vi "CONDOM.vi"() -> ()   [LabVIEW 2018]
panel:
  out "Tank":dbl(slide) scale=0.0..10.0
  in  "Voltage":dbl(knob) scale=0.0..2000.0
  out "Voltage":dbl
  out "Level Lubricante":dbl(slide) scale=0.0..100.0
  in  "Level Lubricante":dbl(knob) scale=0.0..100.0
  out "Lubricante":bool
  in  "Lubricante":bool
  out "MaxLub":bool
  out "MinLub":bool
  out "Lubricante":dbl(slide) scale=0.0..10.0
  out "Voltaje":bool
  in  "Voltaje":bool
  out "LSecado":bool
  in  "Secado":bool
  out "MaxTal":bool
  out "MinTal":bool
  out "LLavado":bool
  in  "Lavado":bool
  out "LTalco":bool
  in  "Talco":bool
  out "Tanque de Talco":dbl(slide) scale=0.0..10.0
  out "MinC":bool
  out "MaxC":bool
  out "Tanque de Condones":dbl(slide) scale=0.0..10.0
  out "L Quitar":bool
  in  "Quitar":bool
  out "T Vulcanus":dbl(slide) scale=0.0..100.0
  in  "T Vulcanus":dbl(knob) scale=0.0..100.0
  out "L Vulcano":bool
  in  "Vulcanizacion":bool
  out "L Bordes":bool
  in  "Bordes":bool
  out "L F2":bool
  in  "Fase2":bool
  out "L F1":bool
  in  "Fase1":bool
  out "LClean":bool
  in  "Clean":bool
  in  "Secadora por Calor":bool
  out "L Seco":bool
  out "T Sec":dbl(slide) scale=0.0..100.0
  in  "T Sec":dbl(knob) scale=0.0..100.0
  out "L Lab":bool
  in  "Lavado":bool
  out "min Lab":bool
  out "Max Lab":bool
  out "Min Bat":bool
  out "Max Bat":bool
  out "min Mad":bool
  out "Max Mad":bool
  out "min4":bool
  out "Max4":bool
  out "min3":bool
  out "Max3":bool
  out "min Cal":bool
  out "Max Cal":bool
  out "min Mez":bool
  out "Max Mez":bool
  out "min2":bool
  out "Max2":bool
  out "min1":bool
  out "Max1":bool
  in  "stop":bool
  out "L Cal":bool
  in  "Calentador":bool
  out "CAL":dbl(slide) scale=0.0..150.0
  in  "CAL":dbl(knob) scale=0.0..150.0
  out "Valvula Calentador":bool
  out "Lavado":dbl(slide) scale=0.0..10.0
  out "Calentador":dbl(slide) scale=0.0..10.0
  out "Valvula HOT":bool
  out "Valvula Madu":bool
  out "Valvula Mix":bool
  out "Valvula Agua":bool
  out "Valvula Quimicos":bool
  out "Valvula Jabon":bool
  out "Valvula Latex Normal":bool
  out "Valvula Latex Sensitive":bool
  out "TEMP":dbl(slide) scale=0.0..200.0
  in  "TEMP":dbl(knob) scale=0.0..200.0
  out "L Batea":bool
  out "L Madu":bool
  out "L Mix":bool
  in  "Batea":bool
  in  "Maduracion":bool
  in  "Mezcladora":bool
  out "L Latex S":bool
  out "L Latex N":bool
  out "L AguaQJ":bool
  in  "Latex Sensitive":bool
  in  "Latex Normal":bool
  in  "accion":bool
  out "Maduracion":dbl(slide) scale=0.0..50.0
  out "Max":bool
  out "min":bool
  out "Latex Sensitive":dbl(slide) scale=0.0..10.0
  out "Batea":dbl(slide) scale=0.0..50.0
  out "Mezcladora":dbl(slide) scale=0.0..50.0
  out "Agua":dbl(slide) scale=0.0..20.0
  out "Latex Normal":dbl(slide) scale=0.0..10.0
  out "Jabon":dbl(slide) scale=0.0..10.0
  out "Quimicos":dbl(slide) scale=0.0..10.0
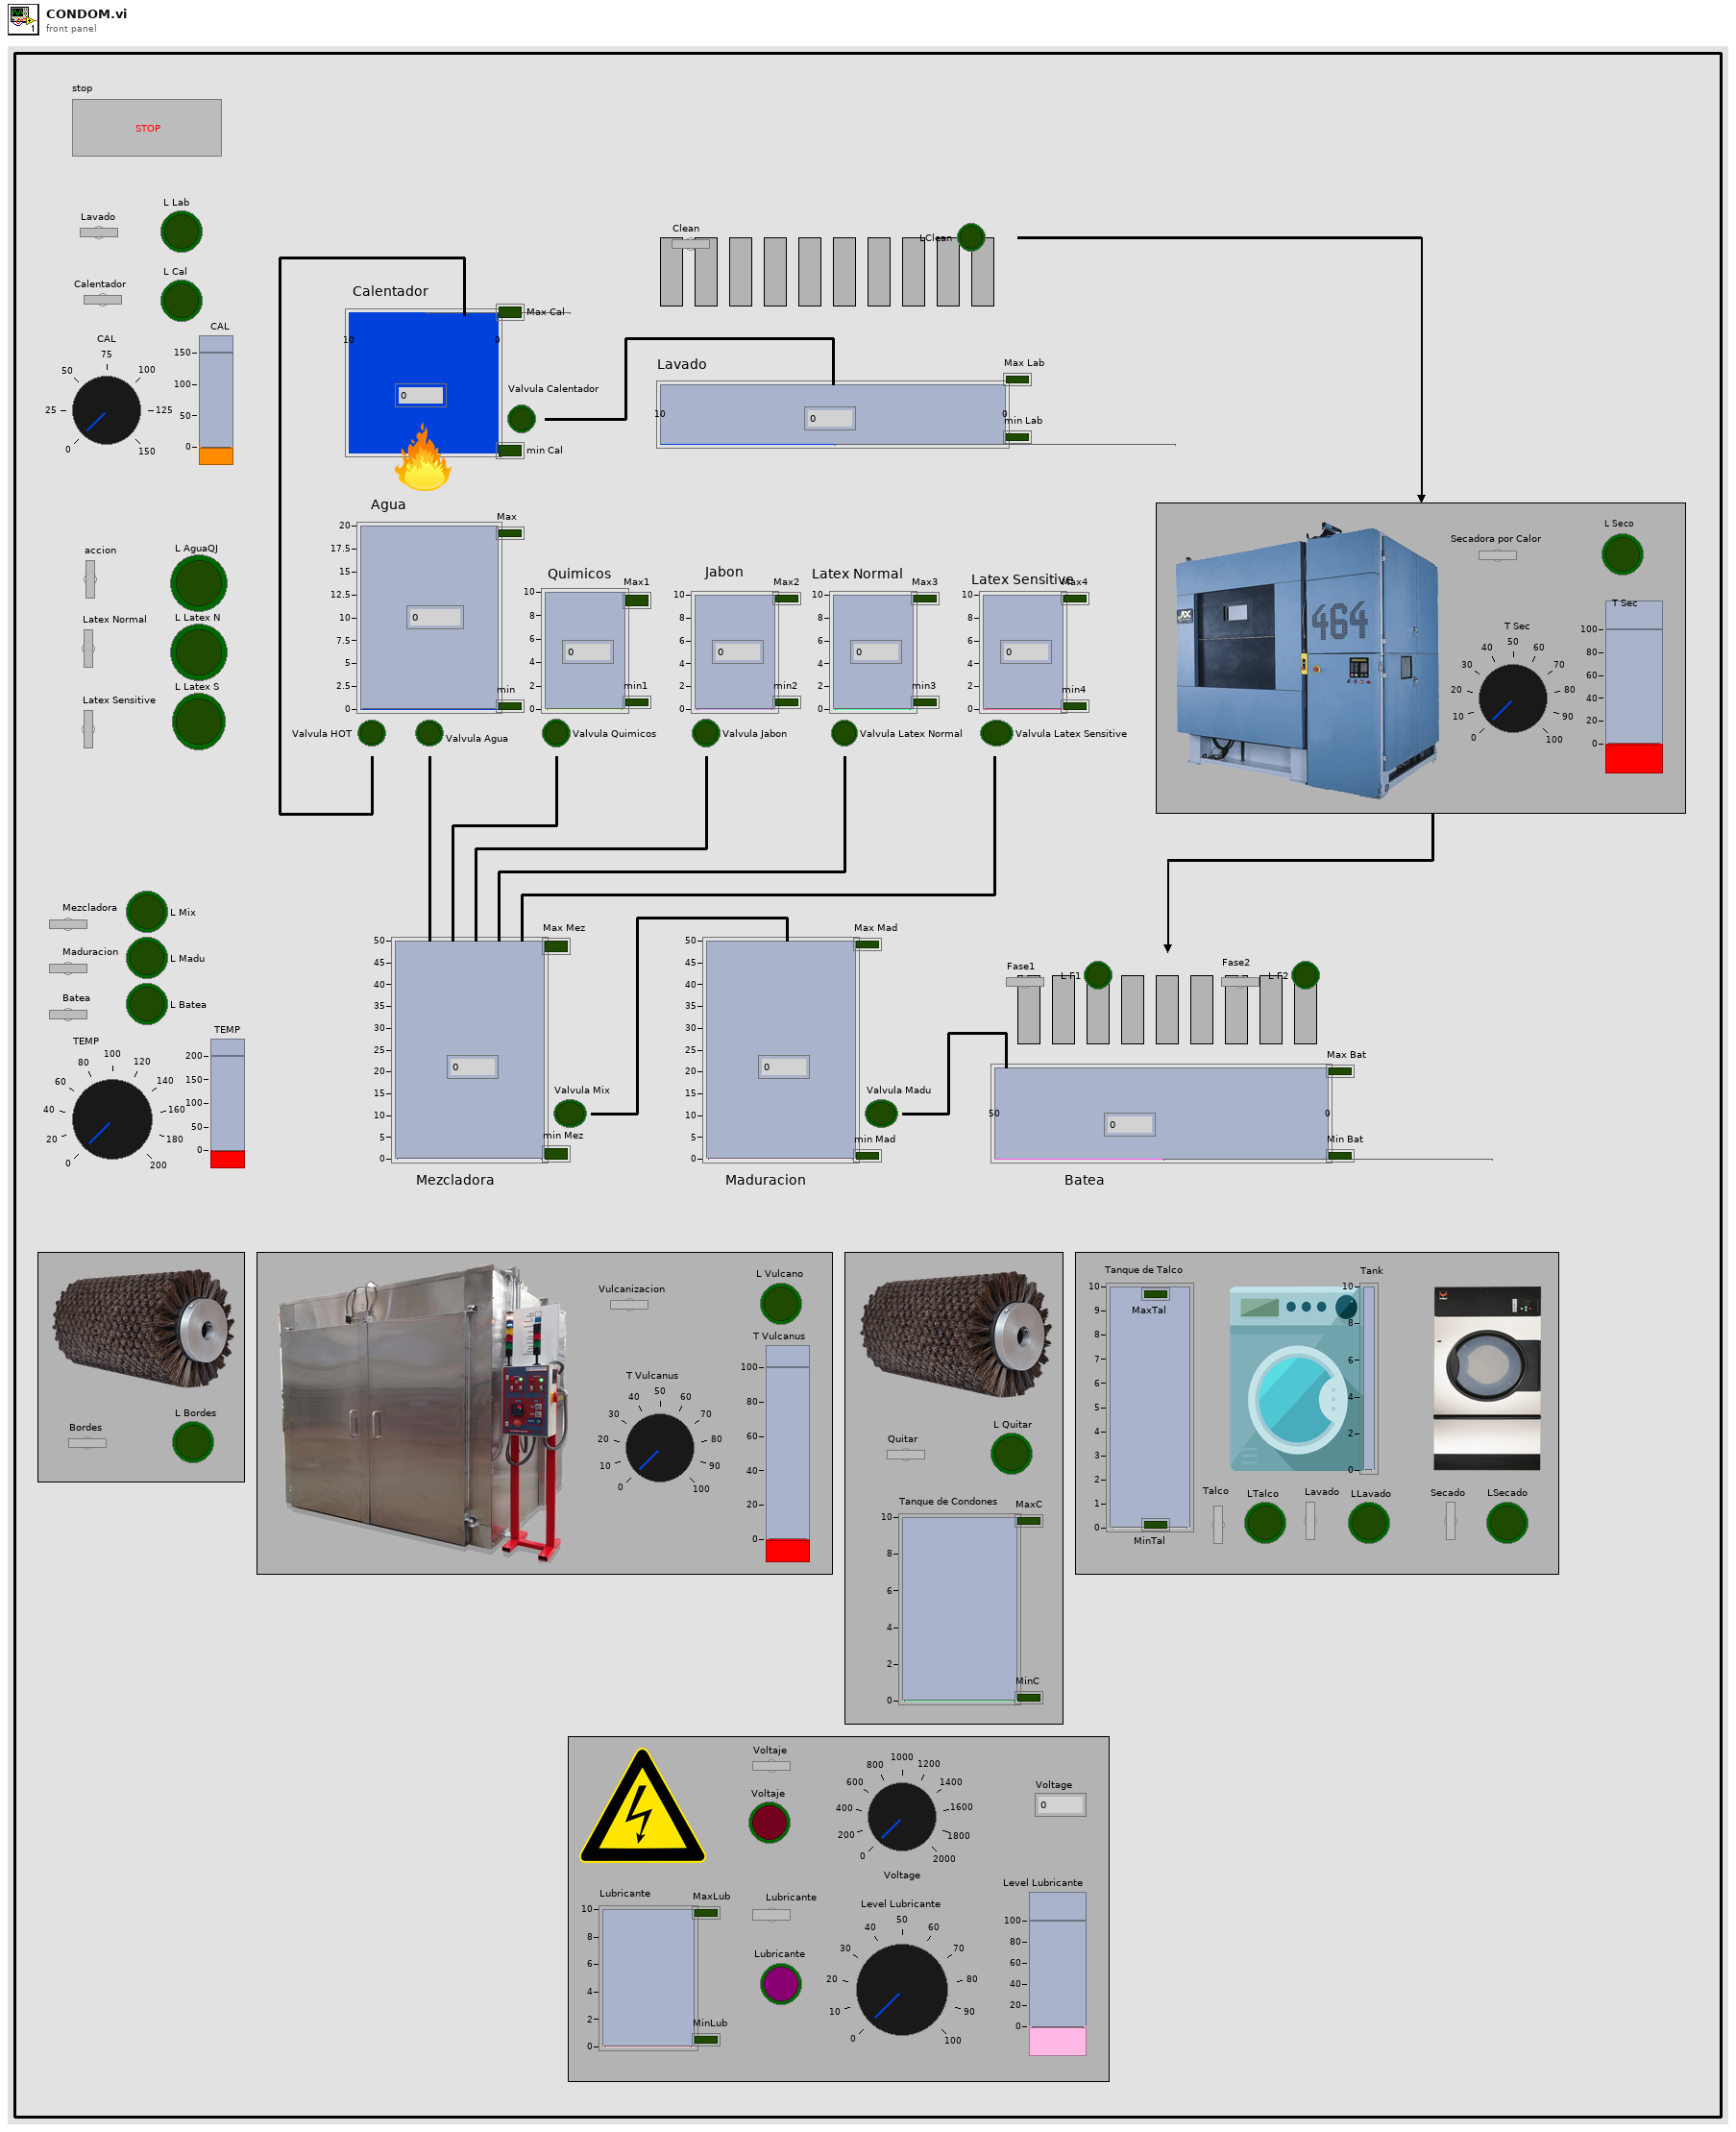
[diagram p1: front panel]
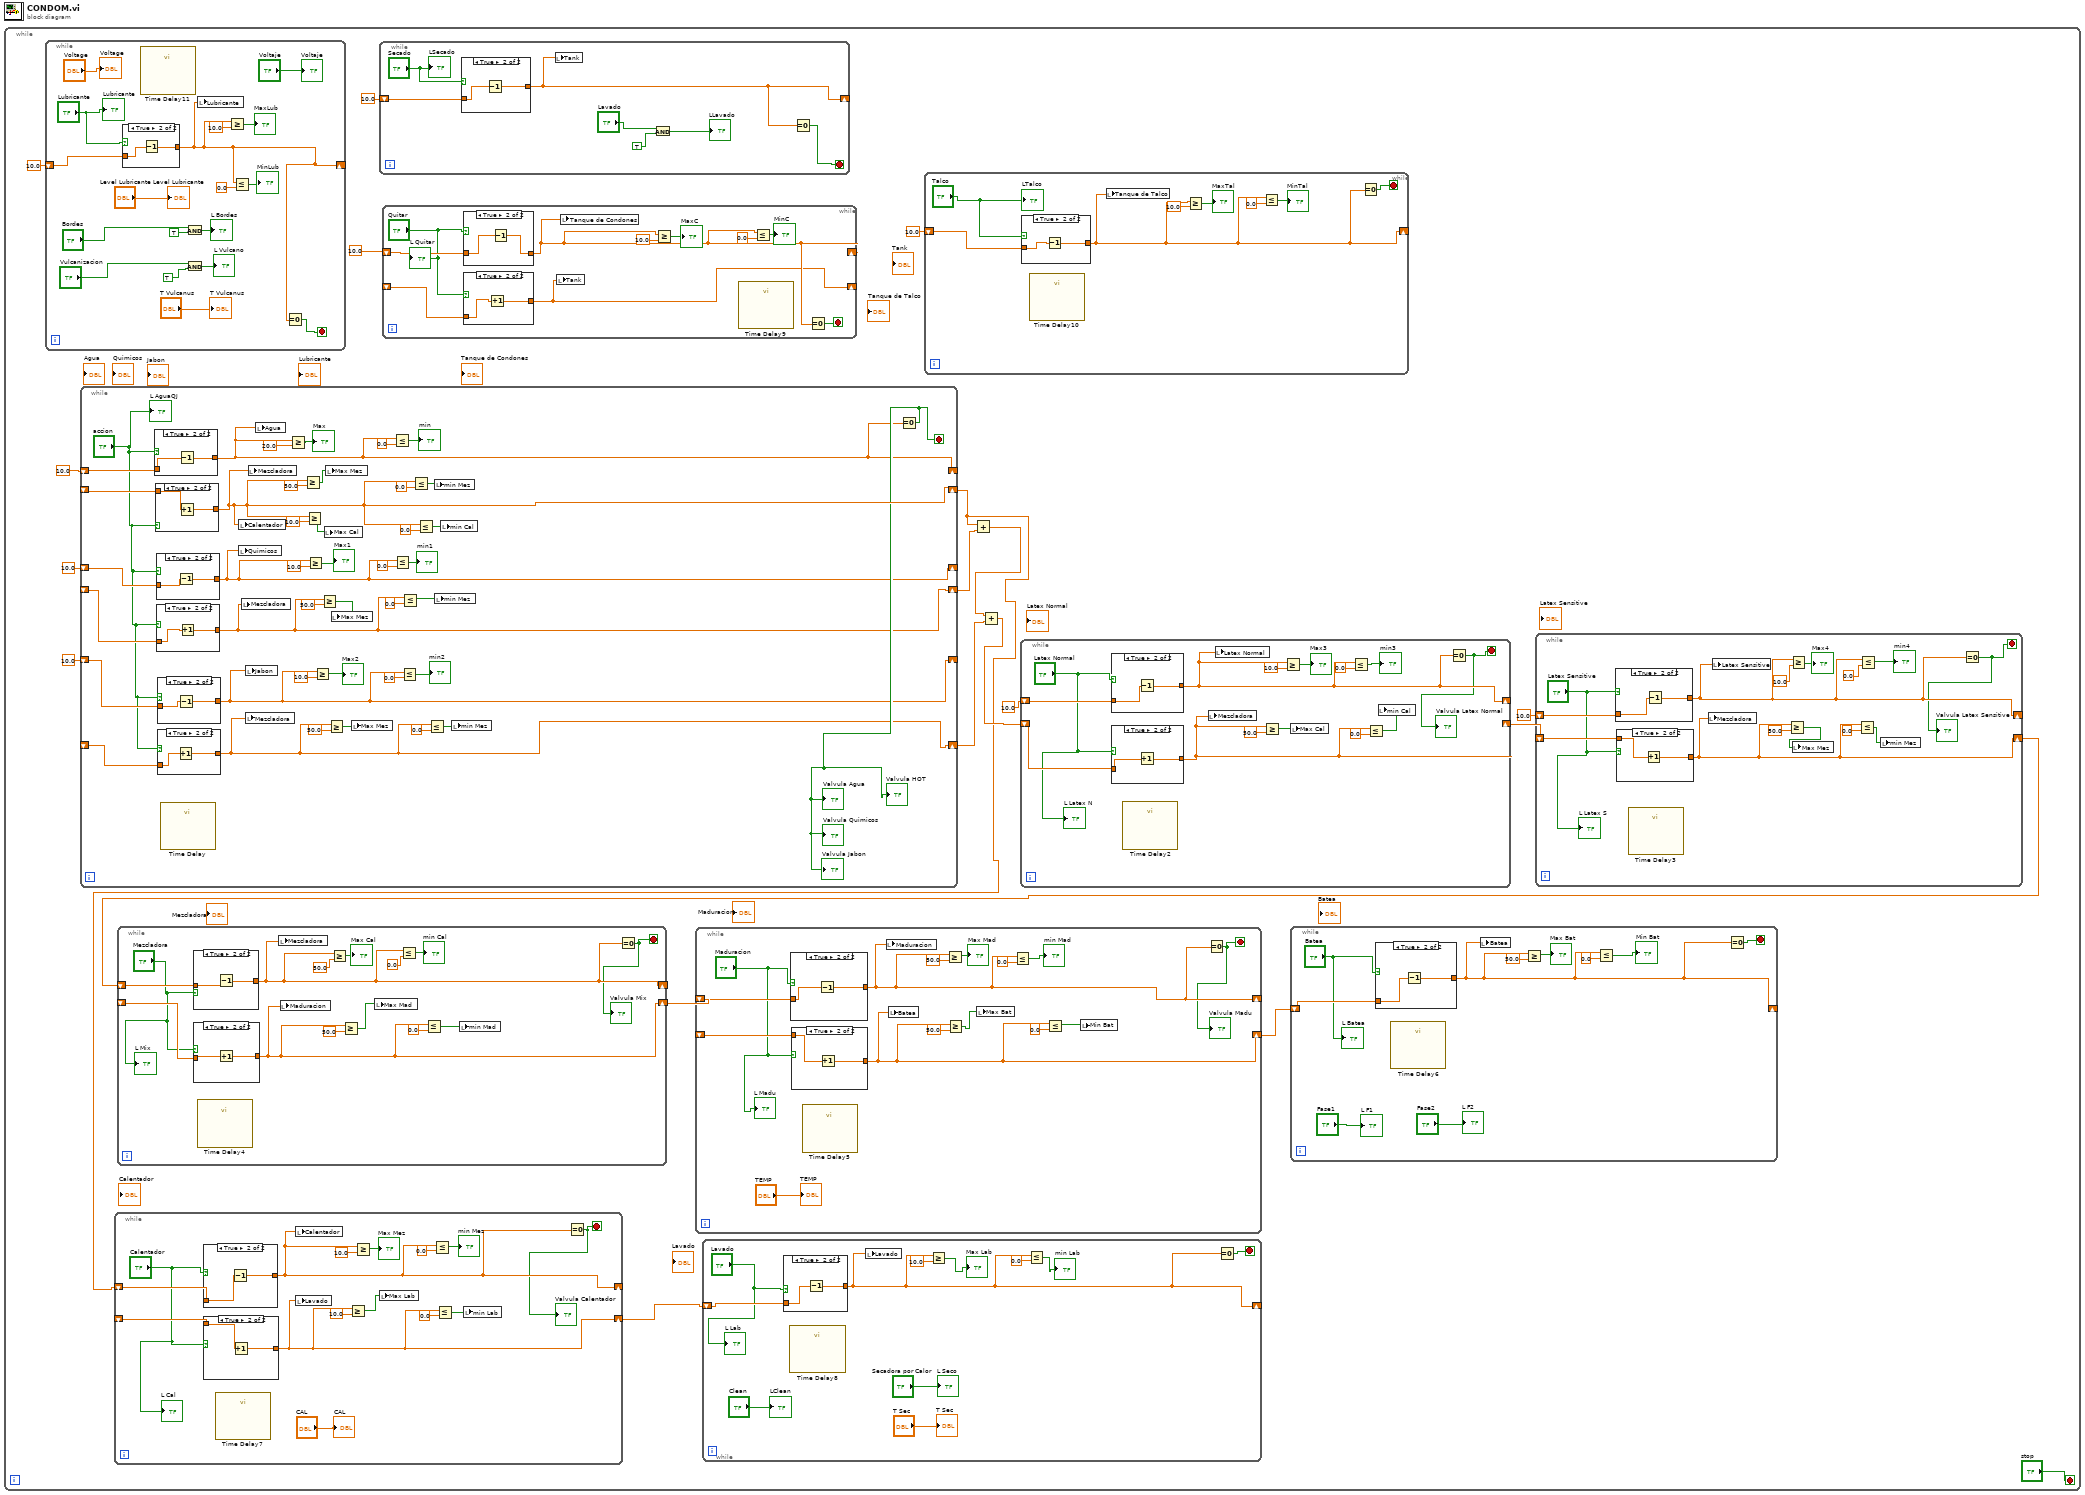
[diagram p0: block diagram]
diagram:
  n1 = while {
    stop <- "stop" stop-if-true
    n2 = while {
      shift-right: [w40] -> _
      shift-left: 10.0 -> [w47]
      stop <- w41 stop-if-true
      n3 = case shown="True" "Lubricante" {
        tunnel: w47 -> [w49 w51]
        tunnel: [w49 w50] -> w40
        frame False {
        }
        frame True {
          n4 = Decrement(x=w51) -> (x-1=w50:dbl)
        }
      }
      n5 = call "Time Delay11"() -> ()  [unwired: 11 in, 1 out]
      n6 = And(x="Bordes", y=TRUE) -> (x .and. y?=→"L Bordes":bool)
      n7 = And(x="Vulcanizacion", y=TRUE) -> (x .and. y?=→"L Vulcano":bool)
      n8 = local write "Lubricante"(w40) -> ()
      n9 = Greater Or Equal?(x=w40, y=10.0) -> (x >= y?=→"MaxLub":bool)
      n10 = Less Or Equal?(x=w40, y=0.0) -> (x <= y?=→"MinLub":bool)
      n11 = Equal To 0?(x=w40) -> (x = 0?=w41:bool)
      "Level Lubricante" <- "Level Lubricante"
      "Lubricante" <- "Lubricante"
      "Voltaje" <- "Voltaje"
      "Voltage" <- "Voltage"
      "T Vulcanus" <- "T Vulcanus"
    }
    n12 = while {
      shift-right: [w219] -> _
      shift-left: 10.0 -> [w229]
      shift-right: [w223] -> w6
      shift-left: _ -> [w228]
      shift-right: [w213] -> _
      shift-left: 10.0 -> [w216]
      shift-right: [w201] -> w10
      shift-left: _ -> [w215]
      shift-right: [w212] -> _
      shift-left: 10.0 -> [w214]
      shift-right: [w193] -> w8
      shift-left: _ -> [w196]
      stop <- w220 stop-if-true
      n13 = case shown="True" "accion" {
        tunnel: w229 -> [w245 w247]
        tunnel: [w245 w246] -> w219
        frame False {
        }
        frame True {
          n14 = Decrement(x=w247) -> (x-1=w246:dbl)
        }
      }
      n15 = case shown="True" "accion" {
        tunnel: w228 -> [w242 w244]
        tunnel: [w242 w243] -> w223
        frame False {
        }
        frame True {
          n16 = Increment(x=w244) -> (x+1=w243:dbl)
        }
      }
      n17 = case shown="True" "accion" {
        tunnel: w216 -> [w239 w241]
        tunnel: [w239 w240] -> w213
        frame False {
        }
        frame True {
          n18 = Decrement(x=w241) -> (x-1=w240:dbl)
        }
      }
      n19 = case shown="True" "accion" {
        tunnel: w215 -> [w236 w238]
        tunnel: [w236 w237] -> w201
        frame False {
        }
        frame True {
          n20 = Increment(x=w238) -> (x+1=w237:dbl)
        }
      }
      n21 = case shown="True" "accion" {
        tunnel: w214 -> [w233 w235]
        tunnel: [w233 w234] -> w212
        frame False {
        }
        frame True {
          n22 = Decrement(x=w235) -> (x-1=w234:dbl)
        }
      }
      n23 = case shown="True" "accion" {
        tunnel: w196 -> [w230 w232]
        tunnel: [w230 w231] -> w193
        frame False {
        }
        frame True {
          n24 = Increment(x=w232) -> (x+1=w231:dbl)
        }
      }
      n25 = call "Time Delay"() -> ()  [unwired: 11 in, 1 out]
      n26 = local write "Calentador"(w223) -> ()
      n27 = local write "Quimicos"(w213) -> ()
      n28 = local write "Mezcladora"(w201) -> ()
      n29 = local write "Mezcladora"(w193) -> ()
      n30 = local write "Jabon"(w212) -> ()
      n31 = local write "Mezcladora"(w223) -> ()
      n32 = local write "Agua"(w219) -> ()
      n33 = Greater Or Equal?(x=w219, y=20.0) -> (x >= y?=→"Max":bool)
      n34 = Greater Or Equal?(x=w223, y=50.0) -> (x >= y?=w203:bool)
      n35 = Greater Or Equal?(x=w223, y=10.0) -> (x >= y?=w189:bool)
      n36 = Greater Or Equal?(x=w213, y=10.0) -> (x >= y?=→"Max1":bool)
      n37 = Greater Or Equal?(x=w212, y=10.0) -> (x >= y?=→"Max2":bool)
      n38 = Greater Or Equal?(x=w201, y=50.0) -> (x >= y?=w198:bool)
      n39 = local write "Max Cal"(w189) -> ()
      n40 = local write "Max Mez"(w203) -> ()
      n41 = Greater Or Equal?(x=w193, y=50.0) -> (x >= y?=w195:bool)
      n42 = local write "Max Mez"(w198) -> ()
      n43 = local write "Max Mez"(w195) -> ()
      n44 = Less Or Equal?(x=w219, y=0.0) -> (x <= y?=→"min":bool)
      n45 = Less Or Equal?(x=w213, y=0.0) -> (x <= y?=→"min1":bool)
      n46 = Less Or Equal?(x=w212, y=0.0) -> (x <= y?=→"min2":bool)
      n47 = Less Or Equal?(x=w201, y=0.0) -> (x <= y?=w197:bool)
      n48 = Less Or Equal?(x=w223, y=0.0) -> (x <= y?=w202:bool)
      n49 = Less Or Equal?(x=w223, y=0.0) -> (x <= y?=w188:bool)
      n50 = Less Or Equal?(x=w193, y=0.0) -> (x <= y?=w194:bool)
      n51 = local write "min Mez"(w202) -> ()
      n52 = local write "min Mez"(w197) -> ()
      n53 = local write "min Cal"(w188) -> ()
      n54 = local write "min Mez"(w194) -> ()
      n55 = Equal To 0?(x=w219) -> (x = 0?=w220:bool)
      "Valvula Agua" <- w220
      "Valvula Jabon" <- w220
      "Valvula Quimicos" <- w220
      "Valvula HOT" <- w220
      "L AguaQJ" <- "accion"
    }
    n56 = while {
      shift-right: [w101] -> _
      shift-left: w6 -> [w106]
      shift-right: [w99] -> w5
      shift-left: _ -> [w105]
      stop <- w100 stop-if-true
      n57 = case shown="True" "Calentador" {
        tunnel: w106 -> [w111 w113]
        tunnel: [w111 w112] -> w101
        frame False {
        }
        frame True {
          n58 = Decrement(x=w113) -> (x-1=w112:dbl)
        }
      }
      n59 = case shown="True" "Calentador" {
        tunnel: w105 -> [w108 w110]
        tunnel: [w108 w109] -> w99
        frame False {
        }
        frame True {
          n60 = Increment(x=w110) -> (x+1=w109:dbl)
        }
      }
      n61 = call "Time Delay7"() -> ()  [unwired: 11 in, 1 out]
      n62 = local write "Calentador"(w101) -> ()
      n63 = local write "Lavado"(w99) -> ()
      n64 = Greater Or Equal?(x=w99, y=10.0) -> (x >= y?=w94:bool)
      n65 = Greater Or Equal?(x=w101, y=10.0) -> (x >= y?=→"Max Mez":bool)
      n66 = local write "Max Lab"(w94) -> ()
      n67 = Less Or Equal?(x=w101, y=0.0) -> (x <= y?=→"min Mez":bool)
      n68 = Less Or Equal?(x=w99, y=0.0) -> (x <= y?=w93:bool)
      n69 = local write "min Lab"(w93) -> ()
      n70 = Equal To 0?(x=w101) -> (x = 0?=w100:bool)
      "Valvula Calentador" <- w100
      "L Cal" <- "Calentador"
      "CAL" <- "CAL"
    }
    n71 = while {
      shift-right: [w21] -> _
      shift-left: 10.0 -> [w23]
      stop <- w22 stop-if-true
      n72 = case shown="True" "Secado" {
        tunnel: w23 -> [w28 w30]
        tunnel: [w28 w29] -> w21
        frame False {
        }
        frame True {
          n73 = Decrement(x=w30) -> (x-1=w29:dbl)
        }
      }
      n74 = local write "Tank"(w21) -> ()
      n75 = And(x="Lavado", y=TRUE) -> (x .and. y?=→"LLavado":bool)
      n76 = Equal To 0?(x=w21) -> (x = 0?=w22:bool)
      "LSecado" <- "Secado"
    }
    n77 = while {
      shift-right: [w67] -> _
      shift-left: 10.0 -> [w68]
      shift-right: [w63] -> _
      shift-left: _ -> [w64]
      stop <- w66 stop-if-true
      n78 = case shown="True" "Quitar" {
        tunnel: w68 -> [w76 w77]
        tunnel: [w76 w78] -> w67
        frame False {
        }
        frame True {
          n79 = Decrement(x=w77) -> (x-1=w78:dbl)
        }
      }
      n80 = case shown="True" "Quitar" {
        tunnel: w64 -> [w73 w75]
        tunnel: [w73 w74] -> w63
        frame False {
        }
        frame True {
          n81 = Increment(x=w75) -> (x+1=w74:dbl)
        }
      }
      n82 = local write "Tank"(w63) -> ()
      n83 = local write "Tanque de Condones"(w67) -> ()
      n84 = Greater Or Equal?(x=w67, y=10.0) -> (x >= y?=→"MaxC":bool)
      n85 = call "Time Delay9"() -> ()  [unwired: 11 in, 1 out]
      n86 = Less Or Equal?(x=w67, y=0.0) -> (x <= y?=→"MinC":bool)
      n87 = Equal To 0?(x=w67) -> (x = 0?=w66:bool)
      "L Quitar" <- "Quitar"
    }
    n88 = while {
      shift-right: [w83] -> _
      shift-left: w5 -> [w89]
      stop <- w82 stop-if-true
      n89 = case shown="True" "Lavado" {
        tunnel: w89 -> [w90 w92]
        tunnel: [w90 w91] -> w83
        frame False {
        }
        frame True {
          n90 = Decrement(x=w92) -> (x-1=w91:dbl)
        }
      }
      n91 = call "Time Delay8"() -> ()  [unwired: 11 in, 1 out]
      n92 = local write "Lavado"(w83) -> ()
      n93 = Greater Or Equal?(x=w83, y=10.0) -> (x >= y?=→"Max Lab":bool)
      n94 = Less Or Equal?(x=w83, y=0.0) -> (x <= y?=→"min Lab":bool)
      n95 = Equal To 0?(x=w83) -> (x = 0?=w82:bool)
      "L Lab" <- "Lavado"
      "LClean" <- "Clean"
      "T Sec" <- "T Sec"
      "L Seco" <- "Secadora por Calor"
    }
    n96 = while {
      shift-right: [w55] -> _
      shift-left: 10.0 -> [w58]
      stop <- w52 stop-if-true
      n97 = case shown="True" "Talco" {
        tunnel: w58 -> [w60 w62]
        tunnel: [w60 w61] -> w55
        frame False {
        }
        frame True {
          n98 = Decrement(x=w62) -> (x-1=w61:dbl)
        }
      }
      n99 = call "Time Delay10"() -> ()  [unwired: 11 in, 1 out]
      n100 = local write "Tanque de Talco"(w55) -> ()
      n101 = Greater Or Equal?(x=w55, y=10.0) -> (x >= y?=→"MaxTal":bool)
      n102 = Less Or Equal?(x=w55, y=0.0) -> (x <= y?=→"MinTal":bool)
      n103 = Equal To 0?(x=w55) -> (x = 0?=w52:bool)
      "LTalco" <- "Talco"
    }
    n104 = Add(x=w6, y=w10) -> (x+y=w9:dbl)
    n105 = Add(x=w9, y=w8) -> (x+y=w7:dbl)
    n106 = while {
      shift-right: [w177] -> _
      shift-left: 10.0 -> [w181]
      shift-right: [w175] -> w17
      shift-left: w7 -> [w180]
      stop <- w176 stop-if-true
      n107 = case shown="True" "Latex Normal" {
        tunnel: w181 -> [w185 w187]
        tunnel: [w185 w186] -> w177
        frame False {
        }
        frame True {
          n108 = Decrement(x=w187) -> (x-1=w186:dbl)
        }
      }
      n109 = case shown="True" "Latex Normal" {
        tunnel: w180 -> [w182 w184]
        tunnel: [w182 w183] -> w175
        frame False {
        }
        frame True {
          n110 = Increment(x=w184) -> (x+1=w183:dbl)
        }
      }
      n111 = call "Time Delay2"() -> ()  [unwired: 11 in, 1 out]
      n112 = local write "Mezcladora"(w175) -> ()
      n113 = local write "Latex Normal"(w177) -> ()
      n114 = Greater Or Equal?(x=w175, y=50.0) -> (x >= y?=w168:bool)
      n115 = Greater Or Equal?(x=w177, y=10.0) -> (x >= y?=→"Max3":bool)
      n116 = local write "Max Cal"(w168) -> ()
      n117 = Less Or Equal?(x=w177, y=0.0) -> (x <= y?=→"min3":bool)
      n118 = Less Or Equal?(x=w175, y=0.0) -> (x <= y?=w169:bool)
      n119 = local write "min Cal"(w169) -> ()
      n120 = Equal To 0?(x=w177) -> (x = 0?=w176:bool)
      "Valvula Latex Normal" <- w176
      "L Latex N" <- "Latex Normal"
    }
    n121 = while {
      shift-right: [w254] -> _
      shift-left: 10.0 -> [w261]
      shift-right: [w257] -> w16
      shift-left: w17 -> [w260]
      stop <- w253 stop-if-true
      n122 = case shown="True" "Latex Sensitive" {
        tunnel: w261 -> [w265 w267]
        tunnel: [w265 w266] -> w254
        frame False {
        }
        frame True {
          n123 = Decrement(x=w267) -> (x-1=w266:dbl)
        }
      }
      n124 = case shown="True" "Latex Sensitive" {
        tunnel: w260 -> [w262 w264]
        tunnel: [w262 w263] -> w257
        frame False {
        }
        frame True {
          n125 = Increment(x=w264) -> (x+1=w263:dbl)
        }
      }
      n126 = call "Time Delay3"() -> ()  [unwired: 11 in, 1 out]
      n127 = local write "Mezcladora"(w257) -> ()
      n128 = local write "Latex Sensitive"(w254) -> ()
      n129 = Greater Or Equal?(x=w257, y=50.0) -> (x >= y?=w248:bool)
      n130 = Greater Or Equal?(x=w254, y=10.0) -> (x >= y?=→"Max4":bool)
      n131 = local write "Max Mez"(w248) -> ()
      n132 = Less Or Equal?(x=w257, y=0.0) -> (x <= y?=w249:bool)
      n133 = Less Or Equal?(x=w254, y=0.0) -> (x <= y?=→"min4":bool)
      n134 = local write "min Mez"(w249) -> ()
      n135 = Equal To 0?(x=w254) -> (x = 0?=w253:bool)
      "Valvula Latex Sensitive" <- w253
      "L Latex S" <- "Latex Sensitive"
    }
    n136 = while {
      shift-right: [w156] -> _
      shift-left: w16 -> [w161]
      shift-right: [w155] -> w15
      shift-left: _ -> [w160]
      stop <- w152 stop-if-true
      n137 = case shown="True" "Mezcladora" {
        tunnel: w161 -> [w165 w167]
        tunnel: [w165 w166] -> w156
        frame False {
        }
        frame True {
          n138 = Decrement(x=w167) -> (x-1=w166:dbl)
        }
      }
      n139 = case shown="True" "Mezcladora" {
        tunnel: w160 -> [w162 w164]
        tunnel: [w162 w163] -> w155
        frame False {
        }
        frame True {
          n140 = Increment(x=w164) -> (x+1=w163:dbl)
        }
      }
      n141 = call "Time Delay4"() -> ()  [unwired: 11 in, 1 out]
      n142 = local write "Mezcladora"(w156) -> ()
      n143 = local write "Maduracion"(w155) -> ()
      n144 = Greater Or Equal?(x=w156, y=50.0) -> (x >= y?=→"Max Cal":bool)
      n145 = Greater Or Equal?(x=w155, y=50.0) -> (x >= y?=w149:bool)
      n146 = local write "Max Mad"(w149) -> ()
      n147 = Less Or Equal?(x=w156, y=0.0) -> (x <= y?=→"min Cal":bool)
      n148 = Less Or Equal?(x=w155, y=0.0) -> (x <= y?=w148:bool)
      n149 = local write "min Mad"(w148) -> ()
      n150 = Equal To 0?(x=w156) -> (x = 0?=w152:bool)
      "Valvula Mix" <- w152
      "L Mix" <- "Mezcladora"
    }
    n151 = while {
      shift-right: [w135] -> _
      shift-left: w15 -> [w141]
      shift-right: [w134] -> w14
      shift-left: _ -> [w140]
      stop <- w131 stop-if-true
      n152 = case shown="True" "Maduracion" {
        tunnel: w141 -> [w145 w147]
        tunnel: [w145 w146] -> w135
        frame False {
        }
        frame True {
          n153 = Decrement(x=w147) -> (x-1=w146:dbl)
        }
      }
      n154 = case shown="True" "Maduracion" {
        tunnel: w140 -> [w142 w144]
        tunnel: [w142 w143] -> w134
        frame False {
        }
        frame True {
          n155 = Increment(x=w144) -> (x+1=w143:dbl)
        }
      }
      n156 = call "Time Delay5"() -> ()  [unwired: 11 in, 1 out]
      n157 = local write "Maduracion"(w135) -> ()
      n158 = local write "Batea"(w134) -> ()
      n159 = Greater Or Equal?(x=w135, y=50.0) -> (x >= y?=→"Max Mad":bool)
      n160 = Greater Or Equal?(x=w134, y=50.0) -> (x >= y?=w127:bool)
      n161 = local write "Max Bat"(w127) -> ()
      n162 = Less Or Equal?(x=w135, y=0.0) -> (x <= y?=→"min Mad":bool)
      n163 = Less Or Equal?(x=w134, y=0.0) -> (x <= y?=w128:bool)
      n164 = local write "Min Bat"(w128) -> ()
      n165 = Equal To 0?(x=w135) -> (x = 0?=w131:bool)
      "Valvula Madu" <- w131
      "L Madu" <- "Maduracion"
      "TEMP" <- "TEMP"
    }
    n166 = while {
      shift-right: [w119] -> _
      shift-left: w14 -> [w123]
      stop <- w118 stop-if-true
      n167 = case shown="True" "Batea" {
        tunnel: w123 -> [w124 w126]
        tunnel: [w124 w125] -> w119
        frame False {
        }
        frame True {
          n168 = Decrement(x=w126) -> (x-1=w125:dbl)
        }
      }
      n169 = call "Time Delay6"() -> ()  [unwired: 11 in, 1 out]
      n170 = local write "Batea"(w119) -> ()
      n171 = Greater Or Equal?(x=w119, y=50.0) -> (x >= y?=→"Max Bat":bool)
      n172 = Less Or Equal?(x=w119, y=0.0) -> (x <= y?=→"Min Bat":bool)
      n173 = Equal To 0?(x=w119) -> (x = 0?=w118:bool)
      "L Batea" <- "Batea"
      "L F1" <- "Fase1"
      "L F2" <- "Fase2"
    }
  }
